vi "Release-timing-source.vi"(8 "error in":errorcluster, 11 "Data ref. in":refnum<data-value>) -> (0 "error IO":errorcluster, 3 "Data ref.":refnum<data-value>)   [LabVIEW 2013, in "CameraVision.lvlib" / "CV-Main.lvclass"]
uses:
  CV-Main.lvclass
  UI/Module-states.ctl
  CV-Main.lvclass/CV-Main.ctl
  Acquisition/CV-Acquisition.lvclass/CV-Acquisition.ctl
  Read Acquis params.vi
  Acquisition/Read Timing source.vi
  Acquisition/Read Gate source.vi
  Acquisition/CV-Acquisition.lvclass
  UI/CV-UI.lvclass
  Errors/CV-Errors.lvclass
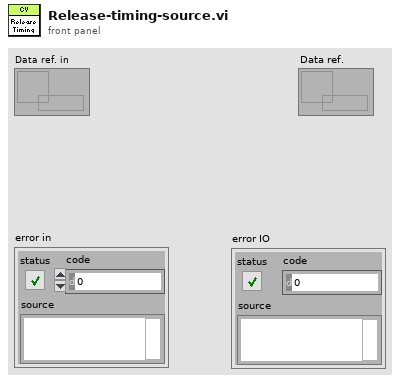
[diagram p1: front panel]
types:
  T1 = typedef "CameraVision.lvlib/CV-UI.lvclass/Module-states.ctl" = enum16{"Inactive", "Active", "Data-loss", "Error", "Simulation", "Synchronizing", "Initialized", "Released"}
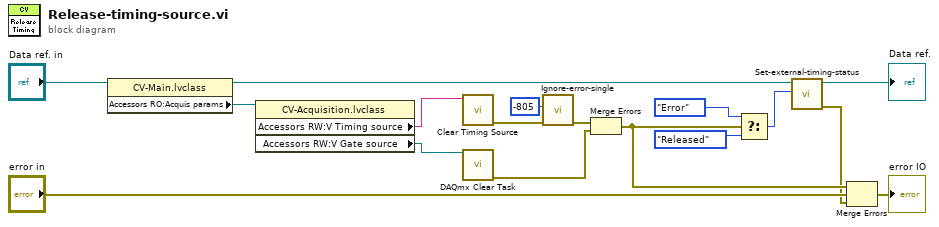
[diagram p0: block diagram]
diagram:
  n1 = property class="CV-Main.lvclass"(reference="Data ref. in") -> (reference out=w9:refnum<data-value>, "Accessors RO:Acquis params"=w14:refnum<data-value>)  [unwired: 1 in, 1 out]
  n2 = property class="CV-Acquisition.lvclass"(reference=w14) -> ("Accessors RW:V Timing source"=w3:string, "Accessors RW:V Gate source"=w13:refnum<k21>)  [unwired: 1 in, 2 out]
  n3 = call <vilib>:"Clear Timing Source.vi"("name"=w3) -> ("error out"=w16:errorcluster)  [unwired: 9 in, 1 out]
  n4 = call <vilib>:"DAQmx Clear Task.vi"("task in"=w13) -> ("error out"=w10:errorcluster)  [unwired: 14 in]
  n5 = call "Ignore-error-single.vi"("error in (no error)"=w16, "Error to ignore"=-805 ("Error to ignore (1)")) -> ("error out"=w11:errorcluster)  [unwired: 9 in]
  n6 = Merge Errors(w11, w10) -> (w6:errorcluster)
  n7 = Select(t=Module-states."Error" ("Acquisition status"), s=w6, f=Module-states."Released" ("Acquisition status")) -> (s? t:f=w7:T1)
  n8 = call "Set-external-timing-status.vi"("Timing status in"=w7, "Data ref. in"=w9) -> ("error IO"=w2:errorcluster, "Data ref."=→"Data ref.":refnum<data-value>)  [unwired: 7 in, 1 out]
  n9 = Merge Errors(w6, "error in", w2) -> (→"error IO":errorcluster)
